vi "Get Display String.vi"(8 "error in (no error)":errorcluster, 11 "FP Equal in":refnum<class "FP Equal.lvclass">) -> (0 "error out":errorcluster, 2 "Display String":string)   [LabVIEW 2018, in "FP Equal.lvclass"]
uses:
  FP Equal.lvclass
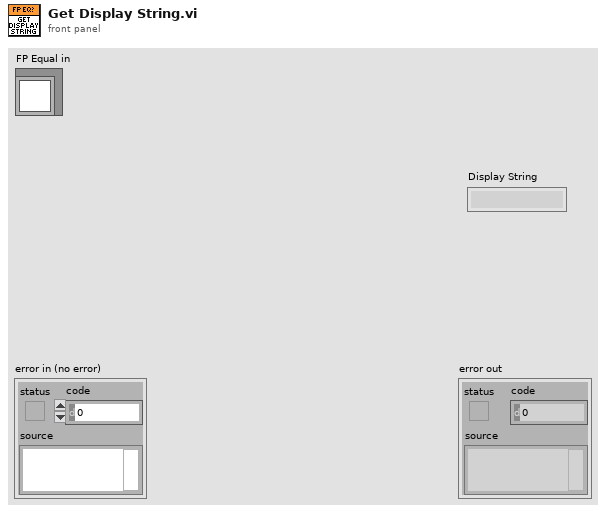
[diagram p1: front panel]
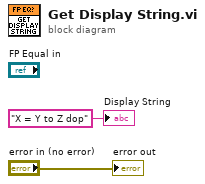
[diagram p0: block diagram]
diagram:
  "error out" <- "error in (no error)"
  "Display String" <- "X = Y to Z dop" ("Display String")
